vi "Training-Master-Slave.vi"() -> ()   [LabVIEW 2016]
doc: "Use this template to build a master/slave design pattern. The master loop always executes. It notifies one or more slave loops to execute their code. The slave loop(s) continue executing until they complete, then wait for another notification. Contrast this with the Producer/Consumer pattern in which the consumer loops execute only when they have data in their queue."
panel:
  out "Stani":bool
  out "Radi":bool
  out "data":dynamicdata(graph)
  out "Slave ITER":i32
  out "Master ITER":i32
  out "Boolean":bool
  out "notification":dbl[](array[numeric])
  in  "Device":u32
  in  "stop":bool
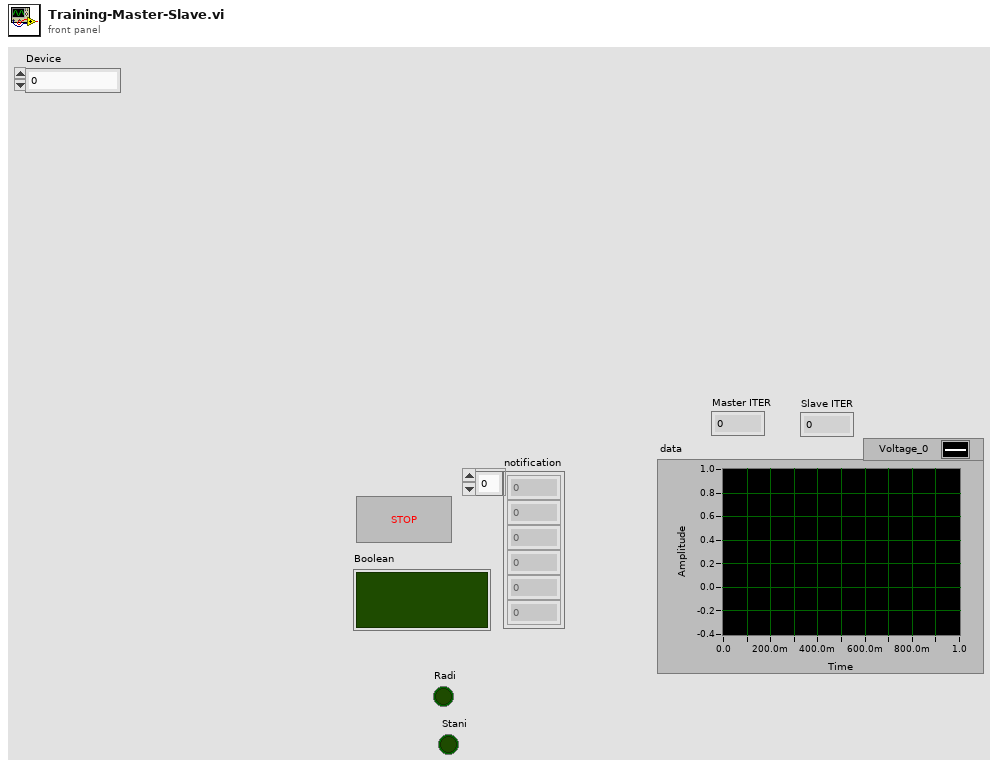
[diagram p1: front panel]
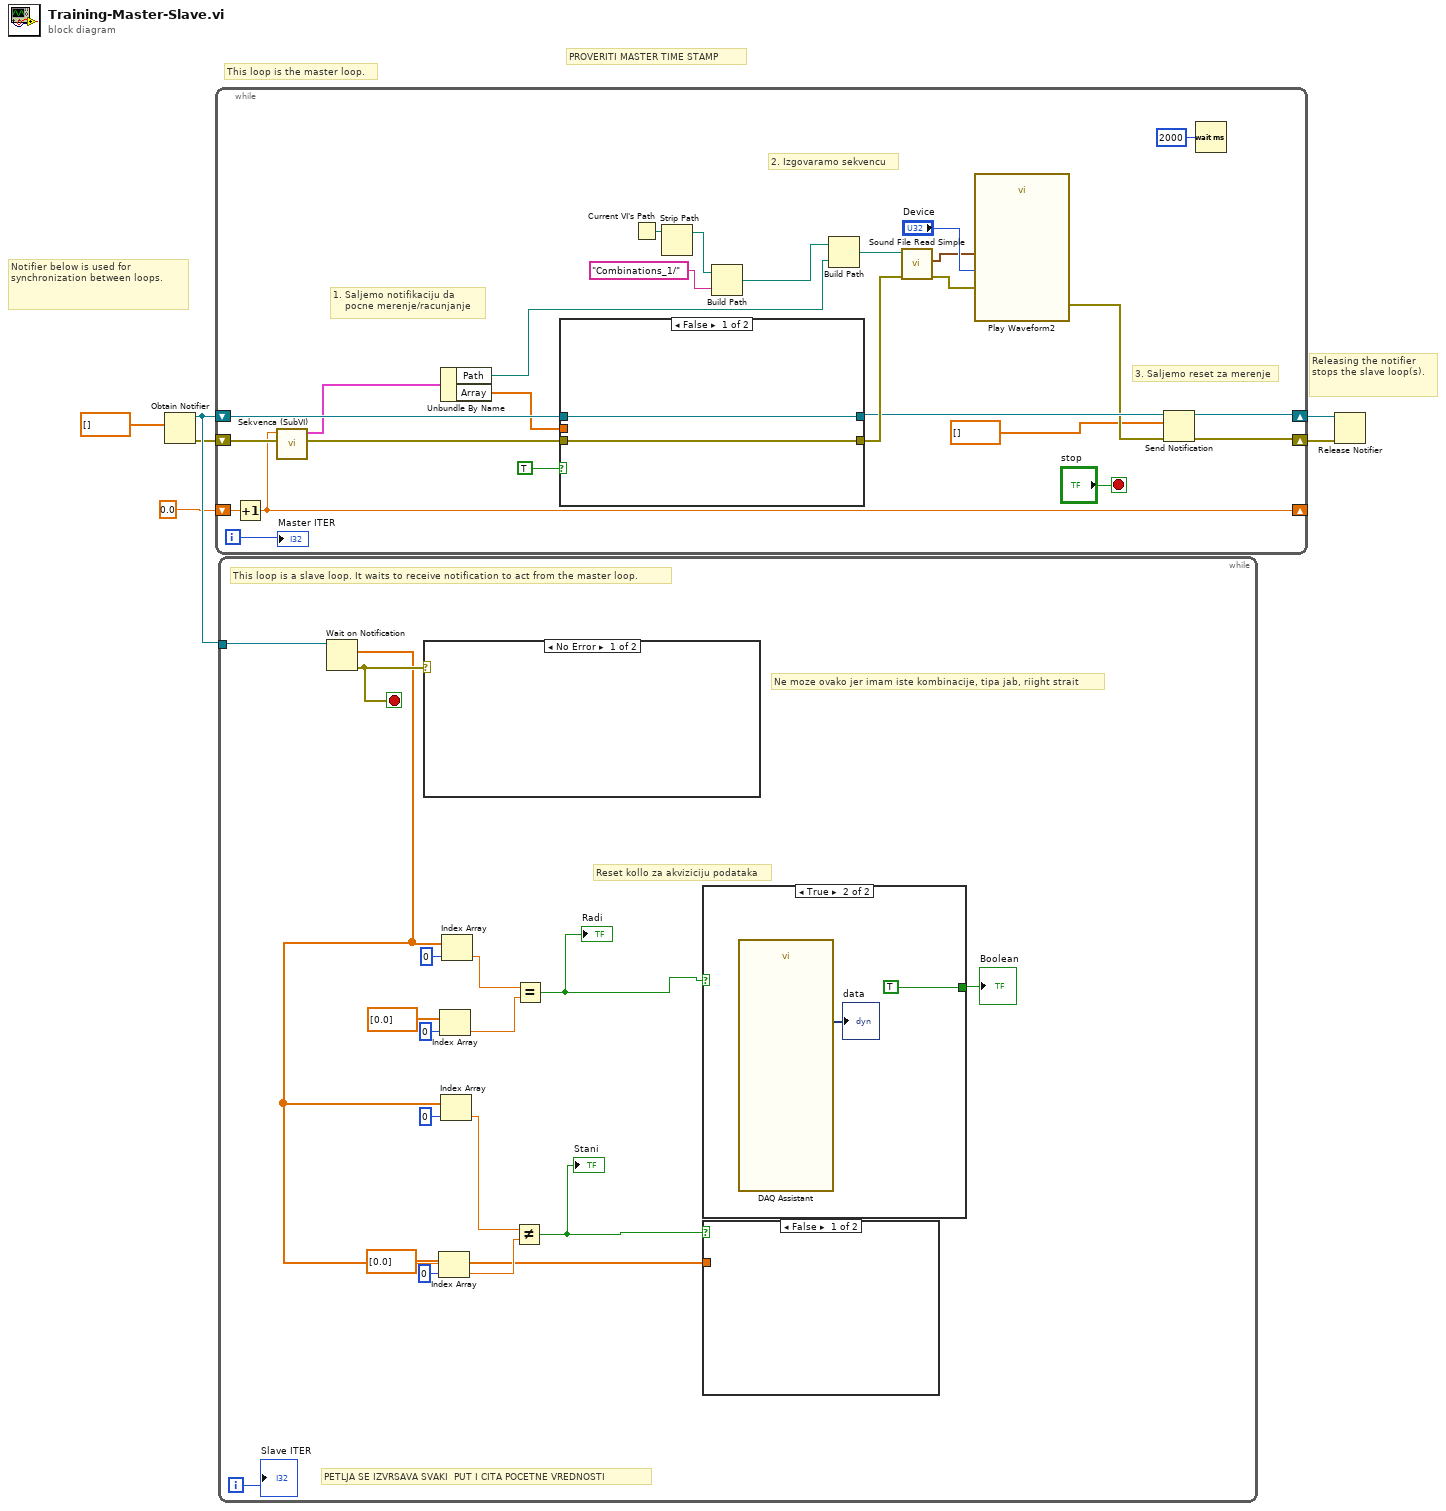
[diagram p0: block diagram]
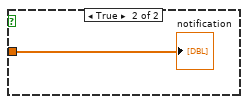
[diagram p2: hidden frame]
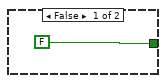
[diagram p3: hidden frame]
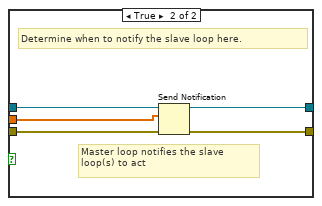
[diagram p5: hidden frame]
diagram:
  # "PROVERITI MASTER TIME STAMP"
  # "This loop is the master loop."
  # "Releasing the notifier stops the slave loop(s)."
  # "Notifier below is used for  synchronization between loops."
  n1 = Obtain Notifier(notification data type=dbl[] [] ("Array")) -> (notifier out=w6:refnum<notifier>, error out=w5:errorcluster)  [unwired: 2 in, 2 out]
  n2 = while {
    shift-right: [w10] -> w4
    shift-left: w5 -> [w29]
    shift-right: [w13] -> w3
    shift-left: w6 -> [w30]
    shift-right: [w27] -> _
    shift-left: 0.0 -> [w28]
    i -> [w7]
    stop <- "stop" stop-if-true
    # "3. Saljemo reset za merenje"
    # "2. Izgovaramo sekvencu"
    # "1. Saljemo notifikaciju da\n    pocne merenje/racunjanje"
    n3 = Increment(x=w28) -> (x+1=w27:dbl)
    n4 = call "Sekvenca (SubVI).vi"("error in (no error)"=w29, "Ulaz"=w27) -> ("error out"=w16:errorcluster, "Cluster 41"=w26:cluster{"Path":path, "Array":dbl[]})  [unwired: 8 in]
    n5 = Unbundle By Name(w26) -> ("Path"=w18:path, "Array"=w17:dbl[])
    n6 = case shown="False" TRUE ("Case Constant\n(See Context Help)") {
      tunnel: w30 -> [w34 w39]
      tunnel: [w33 w38] -> w15
      tunnel: [w34 w37] -> w12
      tunnel: w16 -> [w33 w36]
      tunnel: w17 -> [_ w35]
      frame False {
      }
      frame True {
        # "Determine when to notify the slave loop here."
        # "Master loop notifies the slave loop(s) to act"
        n7 = Send Notification(notification=w35, notifier=w39, error in (no error)=w36) -> (notifier out=w37:refnum<notifier>, error out=w38:errorcluster)
      }
    }
    n8 = Current VI's Path() -> (path=w23:path)
    n9 = Strip Path(path=w23) -> (stripped path=w20:path)  [unwired: 1 out]
    n10 = Build Path(base path=w20, name or relative path="Combinations_1/") -> (appended path=w22:path)
    n11 = Build Path(base path=w22, name or relative path=w18) -> (appended path=w21:path)
    n12 = call <vilib>:"Sound File Read Simple.vi"("error in (no error)"=w15, "path"=w21) -> ("error out"=w25:errorcluster, "data"=w14:waveform(dbl)[])  [unwired: 6 in, 2 out]
    n13 = call "Play Waveform2"("Device"="Device", "Data"=w14, "error in"=w25) -> ("error out"=w11:errorcluster)  [unwired: 16 in]
    n14 = Send Notification(notification=dbl[] [], notifier=w12, error in (no error)=w11) -> (notifier out=w13:refnum<notifier>, error out=w10:errorcluster)
    n15 = Wait (ms)(milliseconds to wait=u32 2000) -> ()  [unwired: 1 out]
    "Master ITER" <- w7
  }
  n16 = while {
    tunnel: w6 -> [w56]
    i -> [w49]
    stop <- w55 stop-if-true
    # "PETLJA SE IZVRSAVA SVAKI  PUT I CITA POCETNE VREDNOSTI"
    # "Reset kollo za akviziciju podataka"
    # "Ne moze ovako jer imam iste kombinacije, tipa jab, riight strait"
    # "This loop is a slave loop. It waits to receive notification to act from the master loop."
    n17 = Wait on Notification(notifier=w56) -> (notification=w43:dbl[], error out=w55:errorcluster)  [unwired: 1 in, 4 out]
    n18 = case shown="No Error" w55 {
      frame No Error {
      }
      frame Error {
      }
    }
    n19 = Index Array(array=dbl[] [0.0] ("notification"), index=0) -> (element=w44:dbl)
    n20 = Index Array(array=dbl[] [0.0] ("notification"), index=0) -> (element=w50:dbl)
    n21 = Index Array(array=w43, index=0) -> (element=w45:dbl)
    n22 = Index Array(array=w43, index=0) -> (element=w51:dbl)
    n23 = Not Equal?(x=w45, y=w44) -> (x != y?=w40:bool)
    "Stani" <- w40
    n24 = Equal?(x=w51, y=w50) -> (x = y?=w41:bool)
    "Radi" <- w41
    n25 = case shown="True" w41 {
      tunnel: [FALSE TRUE] -> w42
      frame False {
      }
      frame True {
        n26 = call "DAQ Assistant"() -> ("data"=→"data":dynamicdata)  [unwired: 16 in, 3 out]
      }
    }
    "Boolean" <- w42
    n27 = case shown="False" w40 {
      tunnel: w43 -> [_ w57]
      frame False {
      }
      frame True {
        "notification" <- w57
      }
    }
    "Slave ITER" <- w49
  }
  n28 = Release Notifier(notifier=w3, error in (no error)=w4) -> ()  [unwired: 4 out]
